vi "rad_Deployment Error Handler.vi"(7 "Deployment Notifiers":T1[](array[typedef]), 8 "error in (no error)":errorcluster[](array[cluster]), 10 "Error Occurred":bool[](array[boolean]), 11 "Queue in":refnum<queue>) -> (0 "error out":errorcluster, 2 "Error Occurred":bool[](array[boolean]), 3 "Queue out":refnum<queue>)   [LabVIEW 2016]
uses:
  TypeDefs/rad_Deployment Notifiers.ctl
  TypeDefs/rad_Deployment Status Data Type.ctl
  TypeDefs/rad_Deployment Progress Data Type.ctl
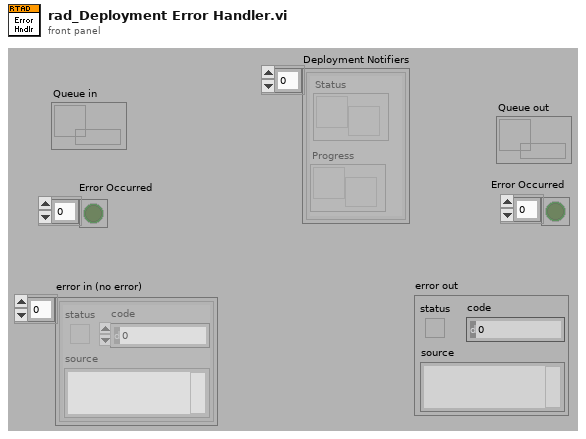
[diagram p1: front panel]
types:
  T1 = typedef "rad_Deployment Notifiers.ctl" = cluster{"Status":refnum<notifier>, "Progress":refnum<notifier>}
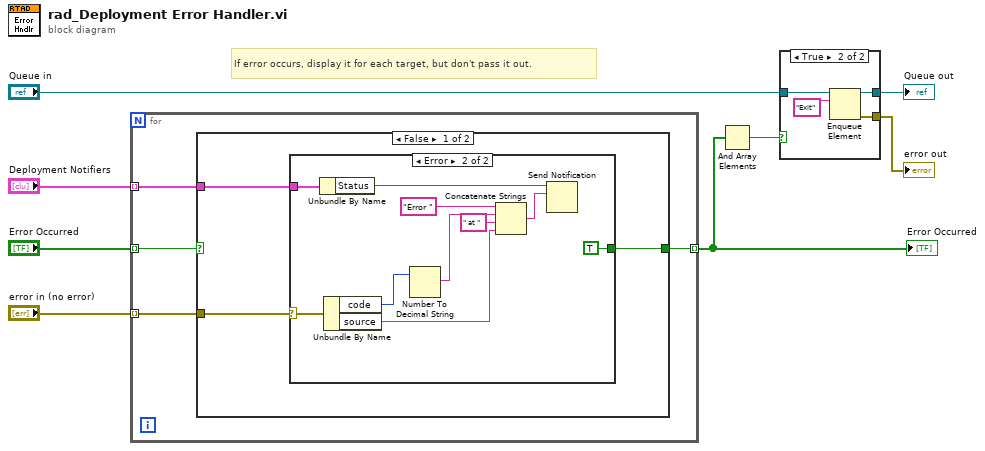
[diagram p0: block diagram]
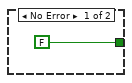
[diagram p3: hidden frame]
diagram:
  # "If error occurs, display it for each target, but don't pass it out."
  n1 = for {
    tunnel: "Error Occurred" -> [w12] mode=indexing
    tunnel: "error in (no error)" -> [w10] mode=indexing
    tunnel: "Deployment Notifiers" -> [w11] mode=indexing
    tunnel: [w9] -> w6 mode=indexing
    n2 = case shown="False" w12 {
      selector: w12 -> [_ w27]
      tunnel: w11 -> [w14 _]
      tunnel: w10 -> [w15 _]
      tunnel: [w13 w27] -> w9
      frame False {
        n3 = case shown="Error" w15 {
          selector: w15 -> [_ w25]
          tunnel: w14 -> [_ w18]
          tunnel: [FALSE TRUE] -> w13
          frame No Error {
          }
          frame Error {
            n4 = Unbundle By Name(w18) -> ("Status"=w17:refnum<notifier>)
            n5 = Unbundle By Name(w25) -> ("code"=w23:i32, "source"=w19:string)
            n6 = Number To Decimal String(number=w23) -> (decimal integer string=w22:string)  [unwired: 1 in]
            n7 = Concatenate Strings("Error " ("string"), w22, " at " ("string"), w19) -> (w21:string)
            n8 = Send Notification(notification=w21, notifier=w17) -> ()  [unwired: 1 in, 2 out]
          }
        }
      }
      frame True {
      }
    }
  }
  "Error Occurred" <- w6
  n9 = And Array Elements(Boolean array=w6) -> (logical AND=w3:bool)
  n10 = case shown="True" w3 {
    tunnel: "Queue in" -> [w28 w32]
    tunnel: [w28 w31] -> w4
    tunnel: [_ w29] -> w2
    frame False {
    }
    frame True {
      n11 = Enqueue Element(queue=w32, element="Exit" ("Message Name")) -> (queue out=w31:refnum<queue>, error out=w29:errorcluster)  [unwired: 2 in, 1 out]
    }
  }
  "error out" <- w2
  "Queue out" <- w4
